vi "Transfer Function Constants.vi"() -> (0 "X":dbl[](array[numeric])=[-1.0, -0.8, -0.7, -0.3, -0.2, 0.0, 0.2, 0.3, 0.7, 0.8, 1.0], 1 "Y":dbl[](array[numeric])=[-1.0, -0.9, -0.85, -0.25, -0.05, 0.0, 0.05, 0.25, 0.85, 0.9, 1.0], 2 "method":i32(ring)=1 items=["nearest", "linear", "spline", "cubic Hermite", "Lagrange"])   [LabVIEW 2011]
doc: "This VI is used as a constant. It will return constant values for the method, the x array, and the y array that are going to be used to interpolate each time it is called. the first time that this VI is called, it will populate front panel graph controls that represent the transform table and the transfer function."
uses:
  <vilib>/gmath/NI_Gmath.lvlib
panel:
  out "Transfer Function":cluster{dbl, dbl}[](graph)=[{-1.0, -1.0}, {-0.99375, -0.996875}, {-0.9875, -0.99375}, {-0.98125, -0.990625}, {-0.975, -0.9875}, {-0.96875, -0.984375}, {-0.9624999999999999, -0.98125}, {-0.9562499999999999, -0.9781249999999999}, {-0.95, -0.975}, {-0.94375, -0.971875}, {-0.9375, -0.96875}, {-0.93125, -0.965625}, {-0.925, -0.9625}, {-0.9187500000000001, -0.9593750000000001}, {-0.9125000000000001, -0.95625}, {-0.90625, -0.953125}, {-0.9, -0.95}, {-0.89375, -0.946875}, {-0.8875, -0.94375}, {-0.88125, -0.940625}, {-0.875, -0.9375}, {-0.86875, -0.934375}, {-0.8625, -0.93125}, {-0.8562500000000001, -0.9281250000000001}, {-0.8500000000000001, -0.925}, {-0.8437500000000001, -0.921875}, {-0.8375000000000001, -0.9187500000000001}, {-0.83125, -0.915625}, {-0.8250000000000001, -0.9125000000000001}, {-0.8187500000000001, -0.909375}, {-0.8125, -0.90625}, {-0.80625, -0.903125}, {-0.8, -0.9}, {-0.796875, -0.8984375}, {-0.7937500000000001, -0.8968750000000001}, {-0.7906250000000001, -0.8953125000000001}, {-0.7875000000000001, -0.89375}, {-0.784375, -0.8921875}, {-0.78125, -0.890625}, {-0.778125, -0.8890625}, {-0.775, -0.8875}, {-0.7718750000000001, -0.8859375}, {-0.76875, -0.884375}, {-0.765625, -0.8828125}, {-0.7625, -0.88125}, {-0.7593749999999999, -0.8796875}, {-0.75625, -0.878125}, {-0.753125, -0.8765625}, {-0.75, -0.875}, {-0.746875, -0.8734375}, {-0.74375, -0.871875}, {-0.7406250000000001, -0.8703125}, {-0.7375, -0.86875}, {-0.734375, -0.8671875}, {-0.73125, -0.865625}, {-0.7281249999999999, -0.8640625}, {-0.725, -0.8625}, {-0.721875, -0.8609375}, {-0.71875, -0.859375}, {-0.715625, -0.8578125}, {-0.7124999999999999, -0.85625}, {-0.7093749999999999, -0.8546874999999999}, {-0.7062499999999999, -0.8531249999999999}, {-0.703125, -0.8515625}, {-0.7, -0.85}, {-0.6875, -0.83125}, {-0.6749999999999999, -0.8125}, {-0.6624999999999999, -0.79375}, {-0.6499999999999999, -0.7749999999999999}, {-0.6375, -0.7562499999999999}, {-0.625, -0.7374999999999999}, {-0.6125, -0.71875}, {-0.6, -0.7}, {-0.5874999999999999, -0.6812499999999999}, {-0.575, -0.6625}, {-0.5625, -0.64375}, {-0.55, -0.625}, {-0.5375000000000001, -0.60625}, {-0.525, -0.5875}, {-0.5125, -0.5687500000000001}, {-0.5, -0.55}, {-0.4875, -0.53125}, {-0.475, -0.5125000000000001}, {-0.4625, -0.49375}, {-0.45, -0.47500000000000003}, {-0.4375, -0.45625000000000004}, {-0.42500000000000004, -0.4375}, {-0.41250000000000003, -0.41875}, {-0.4, -0.4}, {-0.3875, -0.38125000000000003}, {-0.375, -0.36250000000000004}, {-0.3625, -0.34375}, {-0.35, -0.325}, {-0.33749999999999997, -0.30625}, {-0.32499999999999996, -0.2875}, {-0.3125, -0.26875}, {-0.3, -0.25}, {-0.296875, -0.24375000000000002}, {-0.29374999999999996, -0.23749999999999988}, {-0.29062499999999997, -0.2312499999999999}, {-0.2875, -0.22499999999999995}, {-0.284375, -0.21875}, {-0.28125, -0.21250000000000002}, {-0.278125, -0.20625000000000004}, {-0.275, -0.2000000000000001}, {-0.27187500000000003, -0.19375000000000014}, {-0.26875000000000004, -0.18750000000000017}, {-0.265625, -0.18125000000000002}, {-0.2625, -0.17500000000000004}, {-0.259375, -0.16875000000000007}, {-0.25625, -0.16249999999999992}, {-0.253125, -0.15624999999999994}, {-0.25, -0.15}, {-0.246875, -0.14375}, {-0.24375, -0.1375}, {-0.24062499999999998, -0.13125}, {-0.2375, -0.125}, {-0.234375, -0.11875}, {-0.23125, -0.1125}, {-0.22812500000000002, -0.10625000000000001}, {-0.225, -0.1}, {-0.221875, -0.09375}, {-0.21875, -0.08750000000000001}, {-0.215625, -0.08125000000000002}, {-0.21250000000000002, -0.07500000000000001}, {-0.20937500000000003, -0.06875}, {-0.20625000000000002, -0.0625}, {-0.203125, -0.05625}, {-0.2, -0.05}, {-0.19375, -0.0484375}, {-0.1875, -0.046875}, {-0.18125000000000002, -0.045312500000000006}, {-0.17500000000000002, -0.043750000000000004}, {-0.16875, -0.0421875}, {-0.16250000000000003, -0.04062500000000001}, {-0.15625000000000003, -0.03906250000000001}, {-0.15000000000000002, -0.037500000000000006}, {-0.14375000000000002, -0.035937500000000004}, {-0.1375, -0.034375}, {-0.13125, -0.0328125}, {-0.125, -0.03125}, {-0.11875, -0.0296875}, {-0.1125, -0.028125}, {-0.10625000000000001, -0.026562500000000003}, {-0.1, -0.025}, {-0.09375, -0.0234375}, {-0.08750000000000001, -0.021875000000000002}, {-0.08125000000000002, -0.020312500000000004}, {-0.07500000000000001, -0.018750000000000003}, {-0.06875, -0.0171875}, {-0.0625, -0.015625}, {-0.05625, -0.0140625}, {-0.05, -0.0125}, {-0.043750000000000004, -0.010937500000000001}, {-0.037500000000000006, -0.009375000000000001}, {-0.03125, -0.0078125}, {-0.025, -0.00625}, {-0.018750000000000003, -0.004687500000000001}, {-0.0125, -0.003125}, {-0.00625, -0.0015625}, {0.0, 0.0}, {0.00625, 0.0015625}, {0.0125, 0.003125}, {0.018750000000000003, 0.004687500000000001}, {0.025, 0.00625}, {0.03125, 0.0078125}, {0.037500000000000006, 0.009375000000000001}, {0.043750000000000004, 0.010937500000000001}, {0.05, 0.0125}, {0.05625, 0.0140625}, {0.0625, 0.015625}, {0.06875, 0.0171875}, {0.07500000000000001, 0.018750000000000003}, {0.08125000000000002, 0.020312500000000004}, {0.08750000000000001, 0.021875000000000002}, {0.09375, 0.0234375}, {0.1, 0.025}, {0.10625000000000001, 0.026562500000000003}, {0.1125, 0.028125}, {0.11875, 0.0296875}, {0.125, 0.03125}, {0.13125, 0.0328125}, {0.1375, 0.034375}, {0.14375000000000002, 0.035937500000000004}, {0.15000000000000002, 0.037500000000000006}, {0.15625000000000003, 0.03906250000000001}, {0.16250000000000003, 0.04062500000000001}, {0.16875, 0.0421875}, {0.17500000000000002, 0.043750000000000004}, {0.18125000000000002, 0.045312500000000006}, {0.1875, 0.046875}, {0.19375, 0.0484375}, {0.2, 0.05}, {0.203125, 0.05625}, {0.20625000000000002, 0.0625}, {0.20937500000000003, 0.06875}, {0.21250000000000002, 0.07500000000000001}, {0.215625, 0.08125000000000002}, {0.21875, 0.08750000000000001}, {0.221875, 0.09375}, {0.225, 0.1}, {0.22812500000000002, 0.10625000000000001}, {0.23125, 0.1125}, {0.234375, 0.11875}, {0.2375, 0.125}, {0.24062499999999998, 0.13125}, {0.24375, 0.1375}, {0.246875, 0.14375000000000002}, {0.25, 0.15000000000000002}, {0.253125, 0.15625000000000003}, {0.25625, 0.16250000000000003}, {0.259375, 0.16875}, {0.2625, 0.17500000000000002}, {0.265625, 0.18125000000000002}, {0.26875000000000004, 0.1875}, {0.27187500000000003, 0.19375}, {0.275, 0.2}, {0.278125, 0.20625000000000002}, {0.28125, 0.21250000000000002}, {0.284375, 0.21875}, {0.2875, 0.225}, {0.29062499999999997, 0.23125}, {0.29374999999999996, 0.2375}, {0.296875, 0.24375}, {0.3, 0.25}, {0.3125, 0.26875}, {0.32499999999999996, 0.2875}, {0.33749999999999997, 0.30625}, {0.35, 0.325}, {0.3625, 0.34375}, {0.375, 0.36250000000000004}, {0.3875, 0.38125000000000003}, {0.4, 0.4}, {0.41250000000000003, 0.41875}, {0.42500000000000004, 0.4375}, {0.4375, 0.45625000000000004}, {0.45, 0.47500000000000003}, {0.4625, 0.49375}, {0.475, 0.5125000000000001}, {0.4875, 0.53125}, {0.5, 0.55}, {0.5125, 0.5687500000000001}, {0.525, 0.5875}, {0.5375000000000001, 0.60625}, {0.55, 0.625}, {0.5625, 0.64375}, {0.575, 0.6625}, {0.5874999999999999, 0.6812499999999999}, {0.6, 0.7}, {0.6125, 0.71875}, {0.625, 0.7374999999999999}, {0.6375, 0.7562499999999999}, {0.6499999999999999, 0.7749999999999999}, {0.6624999999999999, 0.79375}, {0.6749999999999999, 0.8125}, {0.6875, 0.83125}, {0.7, 0.85}, {0.703125, 0.8515625}, {0.7062499999999999, 0.8531249999999999}, {0.7093749999999999, 0.8546874999999999}, {0.7124999999999999, 0.85625}, {0.715625, 0.8578125}, {0.71875, 0.859375}, {0.721875, 0.8609375}, {0.725, 0.8625}, {0.7281249999999999, 0.8640625000000001}, {0.73125, 0.8656250000000001}, {0.734375, 0.8671875}, {0.7375, 0.86875}, {0.7406250000000001, 0.8703125}, {0.74375, 0.871875}, {0.746875, 0.8734375}, {0.75, 0.875}, {0.753125, 0.8765625}, {0.75625, 0.878125}, {0.7593749999999999, 0.8796875}, {0.7625, 0.88125}, {0.765625, 0.8828125}, {0.76875, 0.8843749999999999}, {0.7718750000000001, 0.8859374999999999}, {0.775, 0.8875}, {0.778125, 0.8890625}, {0.78125, 0.890625}, {0.784375, 0.8921875}, {0.7875000000000001, 0.89375}, {0.7906250000000001, 0.8953125000000001}, {0.7937500000000001, 0.8968750000000001}, {0.796875, 0.8984375}, {0.8, 0.9}, {0.80625, 0.903125}, {0.8125, 0.90625}, {0.8187500000000001, 0.909375}, {0.8250000000000001, 0.9125000000000001}, {0.83125, 0.9156250000000001}, {0.8375000000000001, 0.9187500000000001}, {0.8437500000000001, 0.921875}, {0.8500000000000001, 0.925}, {0.8562500000000001, 0.9281250000000001}, {0.8625, 0.93125}, {0.86875, 0.934375}, {0.875, 0.9375}, {0.88125, 0.940625}, {0.8875, 0.94375}, {0.89375, 0.9468749999999999}, {0.9, 0.95}, {0.90625, 0.953125}, {0.9125000000000001, 0.9562499999999999}, {0.9187500000000001, 0.9593749999999999}, {0.925, 0.9624999999999999}, {0.93125, 0.965625}, {0.9375, 0.96875}, {0.94375, 0.971875}, {0.95, 0.975}, {0.9562499999999999, 0.9781249999999999}, {0.9624999999999999, 0.98125}, {0.96875, 0.984375}, {0.975, 0.9875}, {0.98125, 0.9906250000000001}, {0.9875, 0.99375}, {0.99375, 0.996875}, {1.0, 1.0}]
  out "Transform Table":cluster{dbl, dbl}[](graph)=[{-1.0, -1.0}, {-0.8, -0.9}, {-0.7, -0.85}, {-0.3, -0.25}, {-0.2, -0.05}, {0.0, 0.0}, {0.2, 0.05}, {0.3, 0.25}, {0.7, 0.85}, {0.8, 0.9}, {1.0, 1.0}]
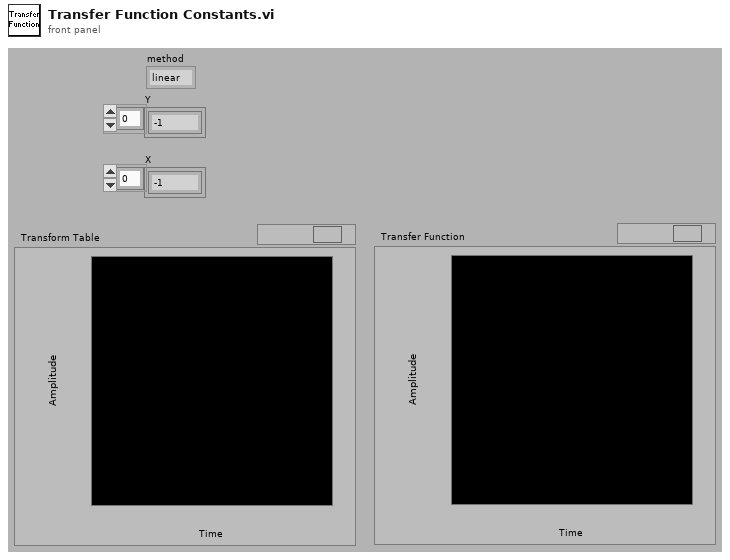
[diagram p1: front panel]
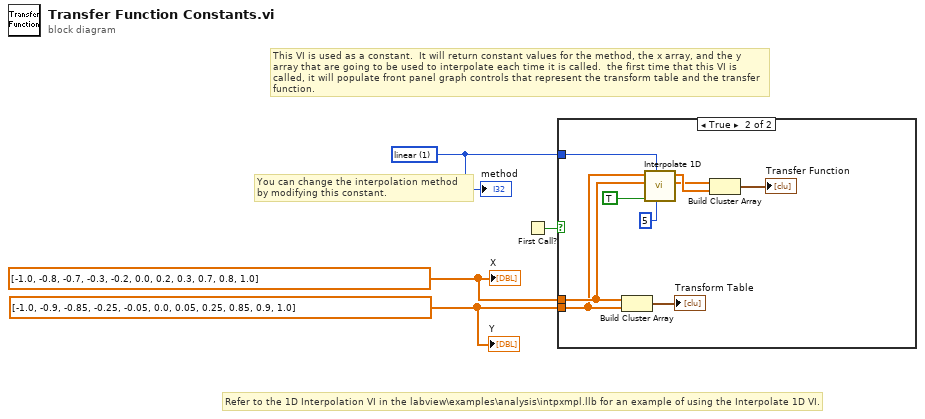
[diagram p0: block diagram]
diagram:
  w3 = 1 items=["nearest", "linear", "spline", "cubic Hermite", "Lagrange"] ("method")
  w2 = dbl[] [-1.0, -0.9, -0.85, -0.25, -0.05, 0.0, 0.05, 0.25, 0.85, 0.9, 1.0]
  w1 = dbl[] [-1.0, -0.8, -0.7, -0.3, -0.2, 0.0, 0.2, 0.3, 0.7, 0.8, 1.0]
  # "You can change the interpolation method\nby modifying this constant."
  # "This VI is used as a constant.  It will return constant values for the method, the x array, and the y array that are going to be used to interpolate each time it is called.  the first time that this VI is called, it will populate front panel graph controls that represent the transform table and the transfer function."
  # "Refer to the 1D Interpolation VI in the labview\\examples\\analysis\\intpxmpl.llb for an example of using the Interpolate 1D VI."
  n1 = First Call?() -> (First Call?: T/F=w4:bool)
  n2 = case shown="True" w4 {
    tunnel: w1 -> [_ w9]
    tunnel: w2 -> [_ w8]
    tunnel: w3 -> [_ w6]
    frame False {
    }
    frame True {
      n3 = Build Cluster Array(w9, w8) -> (→"Transform Table":cluster{dbl, dbl}[])
      n4 = call <vilib>:"Interpolate 1D.vi"("ntimes"=5, "method"=w6, "X is monotonic"=TRUE, "X"=w9, "Y"=w8) -> ("xi used"=w12:dbl[], "yi"=w13:dbl[])  [unwired: 1 in, 4 out]
      n5 = Build Cluster Array(w12, w13) -> (→"Transfer Function":cluster{"Numeric":dbl, "Numeric":dbl}[])
    }
  }
  "Y" <- w2
  "X" <- w1
  "method" <- w3
